vi "multi-function-fpga-Rev4.vi"() -> ()   [LabVIEW 2016]
uses:
  <vilib>/eio/EIONode/EIONode.xnode
  <vilib>/rvi/eio/common/nirviEmuTemplateMethod_errors.vi
  fpga Control.ctl
panel:
  in  "Update":bool
  in  "stop":bool
  in  "fpga controls":T1[](array[typedef]) {"Output - HI" format="%#_17g"; "Output - LO" format="%#_17g"; "Input - B" items=["DIO0", "DIO1", "DIO2", "DIO3", "DIO4", "DIO5", "DIO6", "DIO7", "DIO8", "DIO9", "DIO10", "DIO11", "DIO12", "DIO13", "DIO14", "DIO15", "DIO16", "DIO17", "DIO18", "DIO19", "DIO20", "DIO21", "DIO22", "DIO23", "DIO24", "DIO25", "DIO26", "DIO27", "DIO28", "DIO29", "DIO30", "DIO31"]; "Input - A" items=["DIO0", "DIO1", "DIO2", "DIO3", "DIO4", "DIO5", "DIO6", "DIO7", "DIO8", "DIO9", "DIO10", "DIO11", "DIO12", "DIO13", "DIO14", "DIO15", "DIO16", "DIO17", "DIO18", "DIO19", "DIO20", "DIO21", "DIO22", "DIO23", "DIO24", "DIO25", "DIO26", "DIO27", "DIO28", "DIO29", "DIO30", "DIO31"]; "Step Size" format="%#_17g"; "Begin" format="%#_17g"; "Operation" items=["OFF", "SWITCH", "AND GATE", "OR GATE", "ITERATION"]}
  # "Boolean Operation Outputs"
  # "Iteration Operation Outputs"
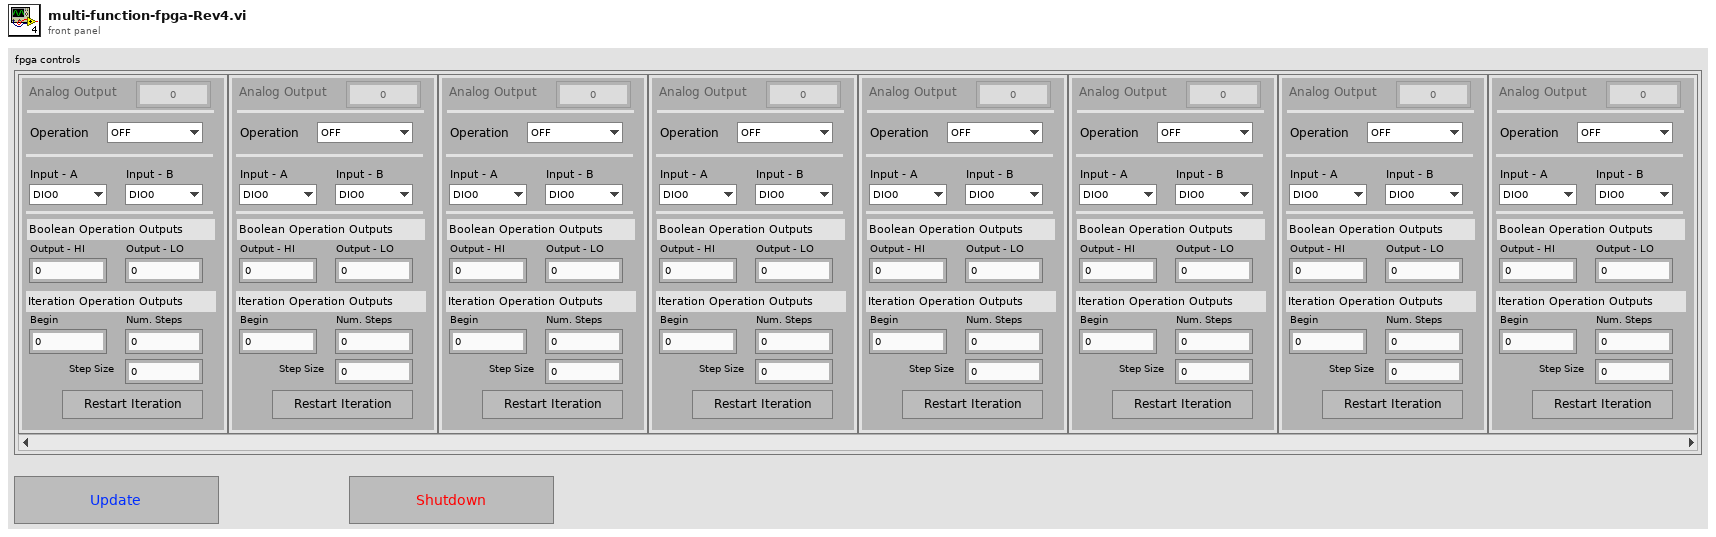
[diagram p1: front panel]
types:
  T1 = typedef "fpga Control.ctl" = cluster{"Operation":i16, "Num. Steps":u16, "Begin":sgl, "Step Size":sgl, "Input - A":i16, "Input - B":i16, "Output - LO":sgl, "Output - HI":sgl, "Reset":bool, "Analog Output":i16}
  T2 = cluster{"[0]":u16, "[1]":u16, "[2]":u16, "[3]":u16, "[4]":u16, "[5]":u16, "[6]":u16, "[7]":u16, "[8]":u16, "[9]":u16, "[10]":u16, "[11]":u16, "[12]":u16, "[13]":u16, "[14]":u16, "[15]":u16}
  T3 = cluster{"[0]":bool, "[1]":bool, "[2]":bool, "[3]":bool, "[4]":bool, "[5]":bool, "[6]":bool, "[7]":bool, "[8]":bool, "[9]":bool, "[10]":bool, "[11]":bool, "[12]":bool, "[13]":bool, "[14]":bool, "[15]":bool}
  T4 = cluster{"fpga controls[0]":T1, "fpga controls[1]":T1, "fpga controls[2]":T1, "fpga controls[3]":T1, "fpga controls[4]":T1, "fpga controls[5]":T1, "fpga controls[6]":T1, "fpga controls[7]":T1, "fpga controls[8]":T1, "fpga controls[9]":T1, "fpga controls[10]":T1, "fpga controls[11]":T1, "fpga controls[12]":T1, "fpga controls[13]":T1, "fpga controls[14]":T1, "fpga controls[15]":T1}
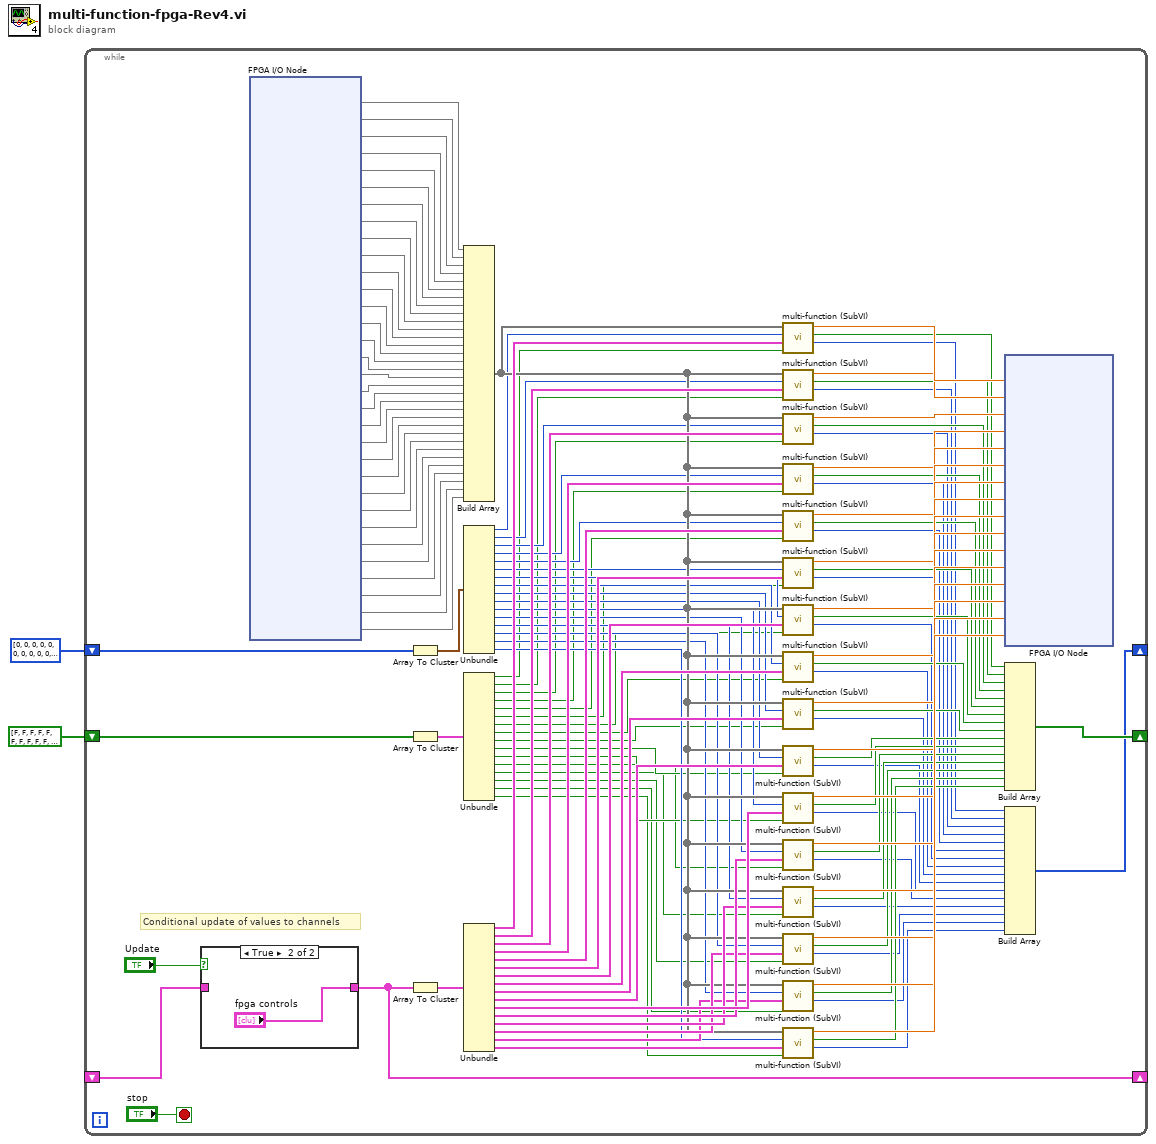
[diagram p0: block diagram]
diagram:
  n1 = while {
    shift-right: [w77] -> _
    shift-left: bool[] [FALSE, FALSE, FALSE, FALSE, FALSE, FALSE, FALSE, FALSE, FALSE, FALSE, FALSE, FALSE, FALSE, FALSE, FALSE, FALSE] -> [w76]
    shift-right: [w7] -> _
    shift-left: u16[] [0, 0, 0, 0, 0, 0, 0, 0, 0, 0, 0, 0, 0, 0, 0, 0] -> [w57]
    shift-right: [w5] -> _
    shift-left: _ -> [w4]
    stop <- "stop" stop-if-true
    # "Conditional update of values to channels"
    n2 = case shown="True" "Update" {
      tunnel: [w143 "fpga controls"] -> w5
      tunnel: w4 -> [w143 _]
      frame False {
      }
      frame True {
      }
    }
    n3 = xnode "FPGA I/O Node"() -> ("Mod2/DIO0"=w142, "Mod2/DIO1"=w141, "Mod2/DIO2"=w140, "Mod2/DIO3"=w139, "Mod2/DIO4"=w138, "Mod2/DIO5"=w137, "Mod2/DIO6"=w136, "Mod2/DIO7"=w135, "Mod2/DIO8"=w134, "Mod2/DIO9"=w133, "Mod2/DIO10"=w132, "Mod2/DIO11"=w131, "Mod2/DIO12"=w130, "Mod2/DIO13"=w129, "Mod2/DIO14"=w128, "Mod2/DIO15"=w127, "Mod2/DIO16"=w126, "Mod2/DIO17"=w125, "Mod2/DIO18"=w124, "Mod2/DIO19"=w123, "Mod2/DIO20"=w122, "Mod2/DIO21"=w121, "Mod2/DIO22"=w120, "Mod2/DIO23"=w119, "Mod2/DIO24"=w118, "Mod2/DIO25"=w117, "Mod2/DIO26"=w116, "Mod2/DIO27"=w115, "Mod2/DIO28"=w114, "Mod2/DIO29"=w113, "Mod2/DIO30"=w112, "Mod2/DIO31"=w111)  [unwired: 32 in, 32 out]
    n4 = Array To Cluster(array=w57) -> (cluster=w56:T2)
    n5 = Array To Cluster(array=w76) -> (cluster=w75:T3)
    n6 = Array To Cluster(array=w5) -> (cluster=w110:T4)
    n7 = Build Array(w142, w141, w140, w139, w138, w137, w136, w135, w134, w133, w132, w131, w130, w129, w128, w127, w126, w125, w124, w123, w122, w121, w120, w119, w118, w117, w116, w115, w114, w113, w112, w111) -> (w58:void[])
    n8 = Unbundle(w56) -> ("[0]"=w55:u16, "[1]"=w54:u16, "[2]"=w53:u16, "[3]"=w52:u16, "[4]"=w51:u16, "[5]"=w50:u16, "[6]"=w49:u16, "[7]"=w48:u16, "[8]"=w47:u16, "[9]"=w46:u16, "[10]"=w45:u16, "[11]"=w44:u16, "[12]"=w43:u16, "[13]"=w42:u16, "[14]"=w41:u16, "[15]"=w40:u16)
    n9 = Unbundle(w75) -> ("[0]"=w39:bool, "[1]"=w38:bool, "[2]"=w37:bool, "[3]"=w36:bool, "[4]"=w35:bool, "[5]"=w34:bool, "[6]"=w33:bool, "[7]"=w32:bool, "[8]"=w31:bool, "[9]"=w30:bool, "[10]"=w29:bool, "[11]"=w28:bool, "[12]"=w27:bool, "[13]"=w26:bool, "[14]"=w25:bool, "[15]"=w24:bool)
    n10 = Unbundle(w110) -> ("fpga controls[0]"=w74:T1, "fpga controls[1]"=w73:T1, "fpga controls[2]"=w72:T1, "fpga controls[3]"=w71:T1, "fpga controls[4]"=w70:T1, "fpga controls[5]"=w69:T1, "fpga controls[6]"=w68:T1, "fpga controls[7]"=w67:T1, "fpga controls[8]"=w66:T1, "fpga controls[9]"=w65:T1, "fpga controls[10]"=w64:T1, "fpga controls[11]"=w63:T1, "fpga controls[12]"=w62:T1, "fpga controls[13]"=w61:T1, "fpga controls[14]"=w60:T1, "fpga controls[15]"=w59:T1)
    n11 = call "multi-function (SubVI).vi"("Step Value Flag In"=w39, "Channel"=w74, "Iter Num In"=w55, "Array"=w58) -> ("Iter Num Out"=w23:u16, "Step Value Flag Out"=w93:bool, "AO out"=w109:sgl)  [unwired: 5 in]
    n12 = call "multi-function (SubVI).vi"("Step Value Flag In"=w38, "Channel"=w73, "Iter Num In"=w54, "Array"=w58) -> ("Iter Num Out"=w22:u16, "Step Value Flag Out"=w92:bool, "AO out"=w108:sgl)  [unwired: 5 in]
    n13 = call "multi-function (SubVI).vi"("Step Value Flag In"=w37, "Channel"=w72, "Iter Num In"=w53, "Array"=w58) -> ("Iter Num Out"=w21:u16, "Step Value Flag Out"=w91:bool, "AO out"=w94:sgl)  [unwired: 5 in]
    n14 = call "multi-function (SubVI).vi"("Step Value Flag In"=w36, "Channel"=w71, "Iter Num In"=w52, "Array"=w58) -> ("Iter Num Out"=w20:u16, "Step Value Flag Out"=w90:bool, "AO out"=w95:sgl)  [unwired: 5 in]
    n15 = call "multi-function (SubVI).vi"("Step Value Flag In"=w35, "Channel"=w70, "Iter Num In"=w51, "Array"=w58) -> ("Iter Num Out"=w19:u16, "Step Value Flag Out"=w89:bool, "AO out"=w96:sgl)  [unwired: 5 in]
    n16 = call "multi-function (SubVI).vi"("Step Value Flag In"=w34, "Channel"=w69, "Iter Num In"=w50, "Array"=w58) -> ("Iter Num Out"=w18:u16, "Step Value Flag Out"=w88:bool, "AO out"=w97:sgl)  [unwired: 5 in]
    n17 = call "multi-function (SubVI).vi"("Step Value Flag In"=w33, "Channel"=w68, "Iter Num In"=w49, "Array"=w58) -> ("Iter Num Out"=w17:u16, "Step Value Flag Out"=w87:bool, "AO out"=w98:sgl)  [unwired: 5 in]
    n18 = call "multi-function (SubVI).vi"("Step Value Flag In"=w32, "Channel"=w67, "Iter Num In"=w48, "Array"=w58) -> ("Iter Num Out"=w16:u16, "Step Value Flag Out"=w86:bool, "AO out"=w99:sgl)  [unwired: 5 in]
    n19 = call "multi-function (SubVI).vi"("Step Value Flag In"=w31, "Channel"=w66, "Iter Num In"=w47, "Array"=w58) -> ("Iter Num Out"=w15:u16, "Step Value Flag Out"=w85:bool, "AO out"=w100:sgl)  [unwired: 5 in]
    n20 = call "multi-function (SubVI).vi"("Step Value Flag In"=w30, "Channel"=w65, "Iter Num In"=w46, "Array"=w58) -> ("Iter Num Out"=w14:u16, "Step Value Flag Out"=w84:bool, "AO out"=w101:sgl)  [unwired: 5 in]
    n21 = call "multi-function (SubVI).vi"("Step Value Flag In"=w29, "Channel"=w64, "Iter Num In"=w45, "Array"=w58) -> ("Iter Num Out"=w13:u16, "Step Value Flag Out"=w83:bool, "AO out"=w102:sgl)  [unwired: 5 in]
    n22 = call "multi-function (SubVI).vi"("Step Value Flag In"=w28, "Channel"=w63, "Iter Num In"=w44, "Array"=w58) -> ("Iter Num Out"=w12:u16, "Step Value Flag Out"=w82:bool, "AO out"=w103:sgl)  [unwired: 5 in]
    n23 = call "multi-function (SubVI).vi"("Step Value Flag In"=w27, "Channel"=w62, "Iter Num In"=w43, "Array"=w58) -> ("Iter Num Out"=w11:u16, "Step Value Flag Out"=w81:bool, "AO out"=w104:sgl)  [unwired: 5 in]
    n24 = call "multi-function (SubVI).vi"("Step Value Flag In"=w26, "Channel"=w61, "Iter Num In"=w42, "Array"=w58) -> ("Iter Num Out"=w10:u16, "Step Value Flag Out"=w80:bool, "AO out"=w105:sgl)  [unwired: 5 in]
    n25 = call "multi-function (SubVI).vi"("Step Value Flag In"=w25, "Channel"=w60, "Iter Num In"=w41, "Array"=w58) -> ("Iter Num Out"=w8:u16, "Step Value Flag Out"=w79:bool, "AO out"=w106:sgl)  [unwired: 5 in]
    n26 = call "multi-function (SubVI).vi"("Step Value Flag In"=w24, "Channel"=w59, "Iter Num In"=w40, "Array"=w58) -> ("Iter Num Out"=w9:u16, "Step Value Flag Out"=w78:bool, "AO out"=w107:sgl)  [unwired: 5 in]
    n27 = xnode "FPGA I/O Node"("Mod4/AO0"=w109, "Mod4/AO1"=w108, "Mod4/AO2"=w94, "Mod4/AO3"=w95, "Mod4/AO4"=w96, "Mod4/AO5"=w97, "Mod4/AO6"=w98, "Mod4/AO7"=w99, "Mod4/AO8"=w100, "Mod4/AO9"=w101, "Mod4/AO10"=w102, "Mod4/AO11"=w103, "Mod4/AO12"=w104, "Mod4/AO13"=w105, "Mod4/AO14"=w106, "Mod4/AO15"=w107) -> ()  [unwired: 16 in, 16 out]
    n28 = Build Array(w93, w92, w91, w90, w89, w88, w87, w86, w85, w84, w83, w82, w81, w80, w79, w78) -> (w77:bool[])
    n29 = Build Array(w23, w22, w21, w20, w19, w18, w17, w16, w15, w14, w13, w12, w11, w10, w8, w9) -> (w7:u16[])
  }
